vi "Largest from Array.vi"(11 "Array":set{string}[](array[numeric])) -> (3 "Largest Network":set{string}(c389))   [LabVIEW 2020, in "NetAn.lvclass"]
uses:
  NetAn.lvclass
  435da730-0d3f-4464-9dd6-06882f9063b6.vi
  <vilib>/Comparison/Less/Less Functor/Less Functor.lvclass
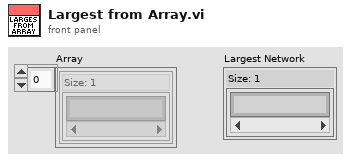
[diagram p1: front panel]
types:
  T1 = cluster{"size":i32, "Largest Network":set{string}}
  T2 = cluster{"size":i32, "Largest Network":set{string}}[]
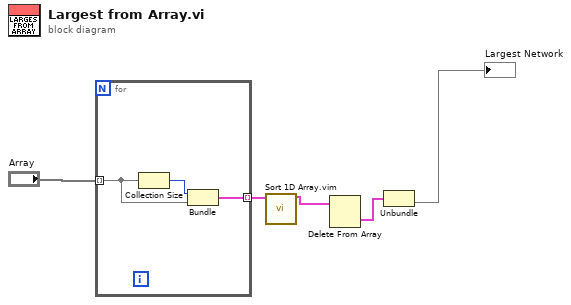
[diagram p0: block diagram]
diagram:
  n1 = for {
    tunnel: "Array" -> [w7] mode=indexing
    tunnel: [w6] -> w2 mode=indexing
    n2 = Collection Size(1:w7) -> (0:w8:i32)
    n3 = Bundle("size"=w8, "Largest Network"=w7) -> (w6:T1)  [unwired: 1 in]
  }
  n4 = call "Sort 1D Array.vim"("unsorted array"=w2) -> ("sorted array"=w3:T2)  [unwired: 10 in]
  n5 = Delete From Array(array=w3) -> (deleted portion=w4:T1)  [unwired: 2 in, 1 out]
  n6 = Unbundle(w4) -> ("Largest Network"=→"Largest Network":set{string})  [unwired: 1 out]
